vi "Loader.vi"(7 "PinMap":path, 8 "error in (no error)":errorcluster, 9 "Pattern Name":string, 10 "BML Frame Array":refnum<class "BML_Frame_Root.lvclass">[](array[class]), 11 "BML_DigiPattern_Generator.lvclass":refnum<class "BML_DigiPattern_Generator.lvclass">) -> (0 "error out":errorcluster, 3 "BML_DigiPattern_Generator.lvclass out":refnum<class "BML_DigiPattern_Generator.lvclass">)   [LabVIEW 2016, in "BML_DigiPattern_Generator.lvclass"]
uses:
  BML_DigiPattern_Generator.lvclass
  BML_Frame_Root/BML_Frame_Root.lvclass
  BML_DigiPattern_Generator.lvclass/BML_DigiPattern_Generator.ctl
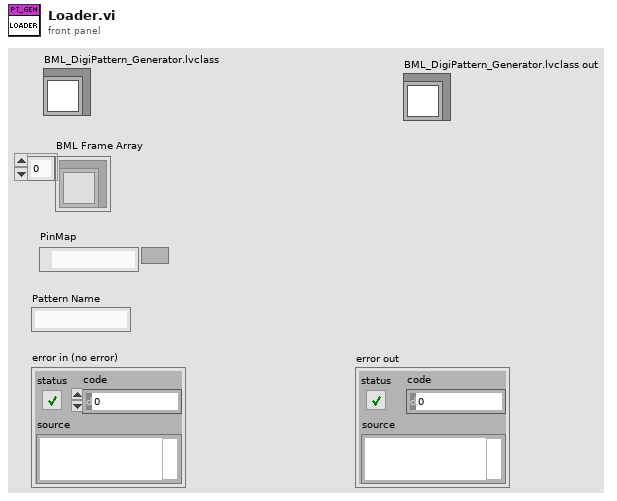
[diagram p1: front panel]
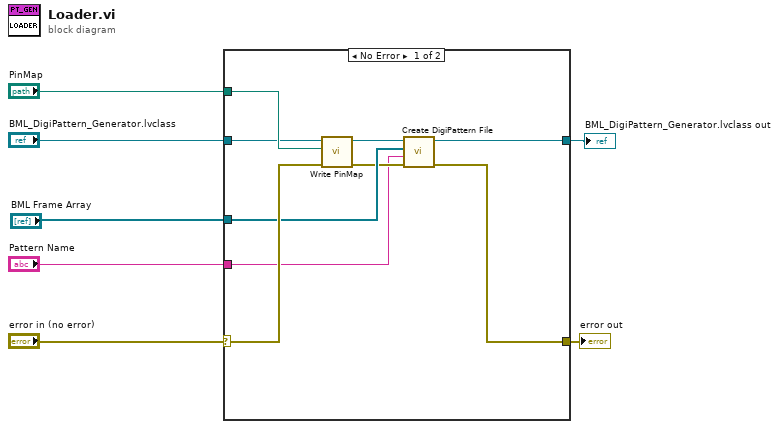
[diagram p0: block diagram]
diagram:
  n1 = case shown="No Error" "error in (no error)" {
    selector: "error in (no error)" -> [w13 w17]
    tunnel: "BML_DigiPattern_Generator.lvclass" -> [w15 w18]
    tunnel: "PinMap" -> [w16 _]
    tunnel: "BML Frame Array" -> [w12 _]
    tunnel: "Pattern Name" -> [w10 _]
    tunnel: [w9 w18] -> w3
    tunnel: [w8 w17] -> w2
    frame No Error {
      n2 = call "Write PinMap.vi"("error in (no error)"=w13, "PinMap"=w16, "BML_DigiPattern_Generator in"=w15) -> ("error out"=w11:errorcluster, "BML_DigiPattern_Generator out"=w14:refnum<class "BML_DigiPattern_Generator.lvclass">)  [unwired: 7 in]
      n3 = call "Create DigiPattern File.vi"("error in (no error)"=w11, "Pattern Name"=w10, "BML Frame Array"=w12, "BML_DigiPattern_Generator.lvclass"=w14) -> ("error out"=w8:errorcluster, "BML_DigiPattern_Generator.lvclass out"=w9:refnum<class "BML_DigiPattern_Generator.lvclass">)  [unwired: 6 in]
    }
    frame Error {
    }
  }
  "BML_DigiPattern_Generator.lvclass out" <- w3
  "error out" <- w2
